vi "Insert Padding.vi"(8 "error in (no error)":errorcluster, 11 "Image":T1) -> (0 "error out":errorcluster, 3 "Image Out":T1)   [LabVIEW 2020, in "G-Image.lvlib"]
uses:
  G-Image.lvlib
  <vilib>/picture/picture.llb/imagedata.ctl
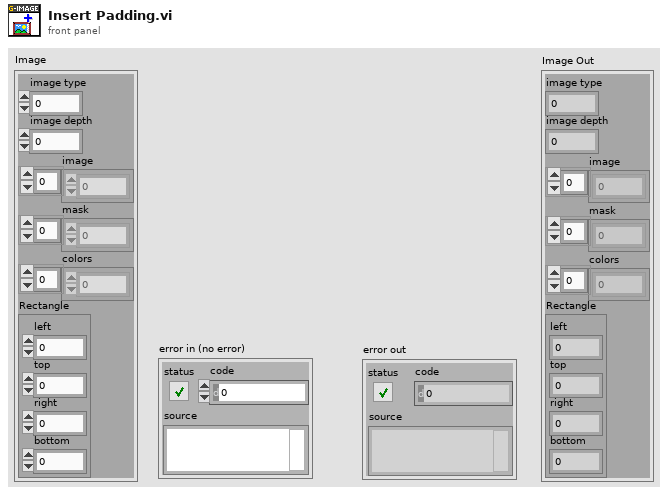
[diagram p1: front panel]
types:
  T1 = typedef "imagedata.ctl" = cluster{"image type":i32, "image depth":i32, "image":u8[], "mask":u8[], "colors":u32[], "Rectangle":cluster{"left":i16, "top":i16, "right":i16, "bottom":i16}}
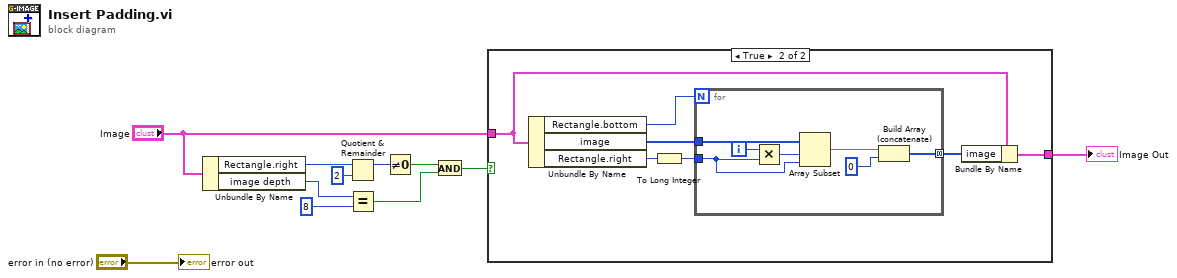
[diagram p0: block diagram]
diagram:
  n1 = Unbundle By Name("Image") -> ("Rectangle.right"=w3:i16, "image depth"=w9:i32)
  n2 = Quotient & Remainder(x=w3, y=i16 2) -> (x-y*floor(x/y)=w7:i16)  [unwired: 1 out]
  n3 = Equal?(x=w9, y=8) -> (x = y?=w5:bool)
  n4 = Not Equal To 0?(x=w7) -> (x != 0?=w6:bool)
  n5 = And(x=w6, y=w5) -> (x .and. y?=w4:bool)
  n6 = case shown="True" w4 {
    tunnel: "Image" -> [w12 w15]
    tunnel: [w12 w13] -> w1
    frame False {
    }
    frame True {
      n7 = Unbundle By Name(w15) -> ("Rectangle.bottom"=w19:i16, "image"=w18:u8[], "Rectangle.right"=w17:i16)
      n8 = To Long Integer(number=w17) -> (32bit integer=w16:i32)
      n9 = for {
        N: w19 -> [_]
        tunnel: w18 -> [w26]
        tunnel: w16 -> [w20]
        tunnel: [w23] -> w14 mode=concatenating
        i -> [w22]
        n10 = Multiply(x=w22, y=w20) -> (x*y=w21:i32)
        n11 = Array Subset(array=w26, index=w21, length=w20) -> (w25:u8[])
        n12 = Build Array (concatenate)(w25, u8 0) -> (w23:u8[])
      }
      n13 = Bundle By Name(cluster=w15, "image"=w14) -> (w13:T1)
    }
  }
  "Image Out" <- w1
  "error out" <- "error in (no error)"
